vi "SelectFormatFile.vi"(8 "error in (no error)":errorcluster, 10 "Forma":enum16{"txt", "CSV"}(ring), 11 "GUI Actor in":refnum<class "GUI Actor.lvclass">) -> (0 "error out":errorcluster, 3 "GUI Actor out":refnum<class "GUI Actor.lvclass">)   [LabVIEW 2019, in "GUI Actor.lvlib" / "GUI Actor.lvclass"]
uses:
  GUI Actor.lvclass
  C:/Program Files (x86)/National Instruments/LabVIEW 2019/vi.lib/ActorFramework/Actor/Actor.lvclass
  GUI Actor.lvclass/GUI Actor.ctl
  Logging/Logging/Logging.lvclass
  CSVV/CSVV/CSVV.lvclass
  E:/7to semestre/instrumentacion virtual/parcial 2/AFTarea/Logging/Logging/Logging.lvclass
  <vilib>/ActorFramework/Message Enqueuer/Message Enqueuer.lvclass/Message Enqueuer.ctl
  <vilib>/ActorFramework/Message Enqueuer/Enqueue.vi
  <vilib>/ActorFramework/Stop Msg/Stop Msg.lvclass
  C:/Program Files (x86)/National Instruments/LabVIEW 2019/vi.lib/ActorFramework/Message/Message.lvclass
  <vilib>/ActorFramework/Message Priority Queue/Priority Enqueue.vi
  <vilib>/ActorFramework/Actor/Actor.lvclass
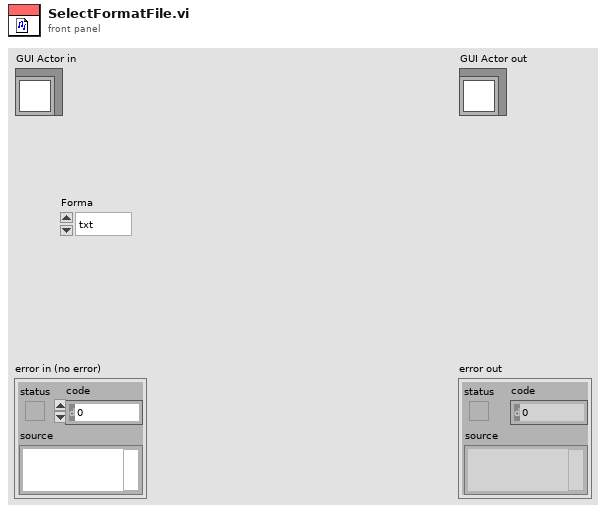
[diagram p1: front panel]
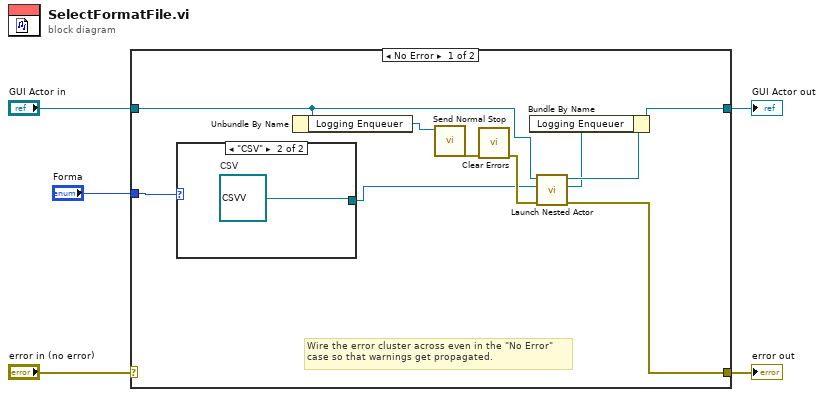
[diagram p0: block diagram]
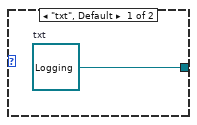
[diagram p2: hidden frame]
diagram:
  n1 = case shown="No Error" "error in (no error)" {
    selector: "error in (no error)" -> [_ w19]
    tunnel: [w8 w19] -> w4
    tunnel: [w14 w18] -> w2
    tunnel: "GUI Actor in" -> [w10 w18]
    tunnel: "Forma" -> [w15 _]
    frame No Error {
      # "Wire the error cluster across even in the \"No Error\"\ncase so that warnings get propagated."
      n2 = case shown="\"CSV\"" w15 {
        tunnel: [w16 w17] -> w7
        frame "txt", Default {
          w16 = refnum<class "Logging.lvclass"> refnum  # txt
        }
        frame "CSV" {
          w17 = refnum<class "CSVV.lvclass"> refnum  # CSV
        }
      }
      n3 = Unbundle By Name(w10) -> ("Logging Enqueuer"=w13:refnum<class "Message Enqueuer.lvclass">)
      n4 = call <vilib>:"Send Normal Stop.vi"("Message Enqueuer"=w13) -> ("error out"=w12:errorcluster)  [unwired: 10 in]
      n5 = call <vilib>:"Clear Errors.vi"("error in (no error)"=w12) -> ("error out"=w11:errorcluster)  [unwired: 5 in, 1 out]
      n6 = call <vilib>:"Launch Nested Actor.vi"("error in (no error)"=w11, "Nested Actor"=w7, "Caller Actor in"=w10) -> ("error out"=w8:errorcluster, "Nested Actor's Enqueuer"=w6:refnum<class "Message Enqueuer.lvclass">, "Caller Actor out"=w9:refnum<class "GUI Actor.lvclass">)  [unwired: 6 in]
      n7 = Bundle By Name(cluster=w9, "Logging Enqueuer"=w6) -> (w14:refnum<class "GUI Actor.lvclass">)
    }
    frame Error {
    }
  }
  "error out" <- w4
  "GUI Actor out" <- w2
